vi "Setup LED Interpolate.vi"(8 "Steps":i32=100, 10 "To":i32 format="%.0x", 11 "From":i32 format="%.0x") -> (3 "Cluster":T1)   [LabVIEW 2014]
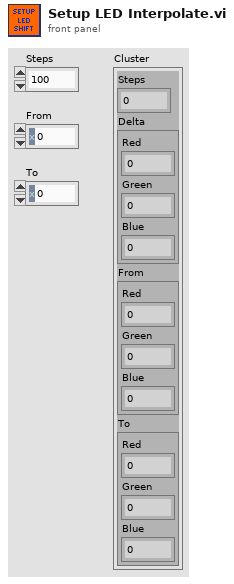
[diagram p1: front panel]
types:
  T1 = cluster{"Steps":i32, "Delta":cluster{"Red":dbl, "Green":dbl, "Blue":dbl}, "From":cluster{"Red":dbl, "Green":dbl, "Blue":dbl}, "To":cluster{"Red":dbl, "Green":dbl, "Blue":dbl}}
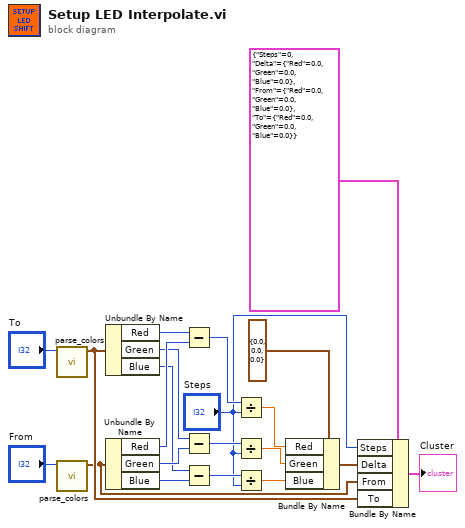
[diagram p0: block diagram]
diagram:
  n1 = call "parse_colors.vi"("Numeric"="To") -> ("Cluster"=w14:cluster{"Red":i32, "Green":i32, "Blue":i32})  [unwired: 10 in]
  n2 = call "parse_colors.vi"("Numeric"="From") -> ("Cluster"=w13:cluster{"Red":i32, "Green":i32, "Blue":i32})  [unwired: 10 in]
  n3 = Unbundle By Name(w14) -> ("Red"=w15:i32, "Green"=w9:i32, "Blue"=w5:i32)
  n4 = Unbundle By Name(w13) -> ("Red"=w16:i32, "Green"=w8:i32, "Blue"=w4:i32)
  n5 = Subtract(x=w15, y=w16) -> (x-y=w17:i32)
  n6 = Subtract(x=w9, y=w8) -> (x-y=w7:i32)
  n7 = Subtract(x=w5, y=w4) -> (x-y=w3:i32)
  n8 = Divide(x=w17, y="Steps") -> (x/y=w19:dbl)
  n9 = Divide(x=w7, y="Steps") -> (x/y=w6:dbl)
  n10 = Divide(x=w3, y="Steps") -> (x/y=w1:dbl)
  n11 = Bundle By Name(cluster=cluster{"Red":dbl, "Green":dbl, "Blue":dbl} {"Red"=0.0, "Green"=0.0, "Blue"=0.0} ("Delta"), "Red"=w19, "Green"=w6, "Blue"=w1) -> (w20:cluster{"Red":dbl, "Green":dbl, "Blue":dbl})
  n12 = Bundle By Name(cluster=T1 {"Steps"=0, "Delta"={"Red"=0.0, "Green"=0.0, "Blue"=0.0}, "From"={"Red"=0.0, "Green"=0.0, "Blue"=0.0}, "To"={"Red"=0.0, "Green"=0.0, "Blue"=0.0}}, "Steps"="Steps", "Delta"=w20, "From"=w13, "To"=w14) -> (→"Cluster":T1)
